vi "User Console View.vi"(8 "error in (no error)":errorcluster, 11 "View Model":T3) -> (0 "error out":errorcluster)   [LabVIEW 2017]
doc: "This console used to select transactions and interact with the ATM controller.\n[Covers: UI2]"
uses:
  View Model/Controls/View Model.ctl
  Error Handler/Controls/Error Model.ctl
  Error Handler/Controls/Error Data.ctl
  Error Handler/Controls/Error Type.ctl
  View Model/Controls/Shared Model.ctl
  Configuration/Controls/Config Model.ctl
  Configuration/Controls/Config CMD.ctl
  Configuration/Controls/Config Data.ctl
  ATM Controller/Controls/Controller Model.ctl
  ATM Controller/Controls/Controller Overhead.ctl
  ATM Controller/Controls/Controller States.ctl
  ATM Controller/Controls/Controller Message Data.ctl
  ATM Controller/Controls/Controller Message Name.ctl
  Controls/User Console - Keypad.ctl
  Controls/User Console - Transactions.ctl
  ATM Controller/Controls/Controller CMD.ctl
panel:
  in  "Card Reader":bool
  in  "Transactions":T1
  in  "Keypad":T2
  # "[Covers: UI2B]"
  # "[Covers: UI2C]"
  # "[Covers: UI2A]"
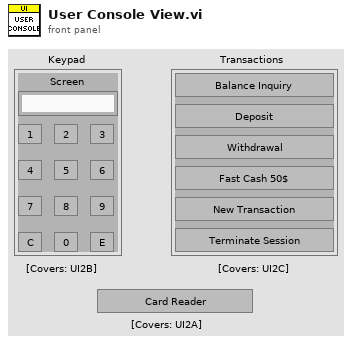
[diagram p1: front panel]
types:
  T1 = typedef "User Console - Transactions.ctl" = cluster{"Balance Inquiry":bool, "Deposit":bool, "Withdrawal":bool, "Fast Cash":bool, "New Transaction":bool, "Terminate":bool}
  T2 = typedef "User Console - Keypad.ctl" = cluster{"Screen":string, "1":bool, "2":bool, "3":bool, "4":bool, "5":bool, "6":bool, "7":bool, "8":bool, "9":bool, "C":bool, "0":bool, "E":bool}
  T3 = typedef "View Model.ctl" = cluster{"Error Model":T4, "Shared Model":T5, "Config Model":T6, "Controller Model":T7}
  T4 = typedef "Error Model.ctl" = cluster{"Error Event":refnum<user-event>}
  T5 = typedef "Shared Model.ctl" = cluster{"Stop Event":refnum<user-event>, "Stop DVR":refnum<data-value>}
  T6 = typedef "Config Model.ctl" = cluster{"Config CMD":refnum<user-event>, "Config Data DVR":refnum<data-value>}
  T7 = typedef "Controller Model.ctl" = cluster{"Controller Overhead DVR":refnum<data-value>, "Deposit Received Change":refnum<user-event>, "Fund Transaction Change":refnum<user-event>, "Card Read Change":refnum<user-event>, "Keypad Change":refnum<user-event>, "Transaction Change":refnum<user-event>, "Controller CMD Change":refnum<user-event>, "Message Change":refnum<user-event>}
  T8 = enum8{"Enabled", "Disabled", "Disabled and Grayed Out"}
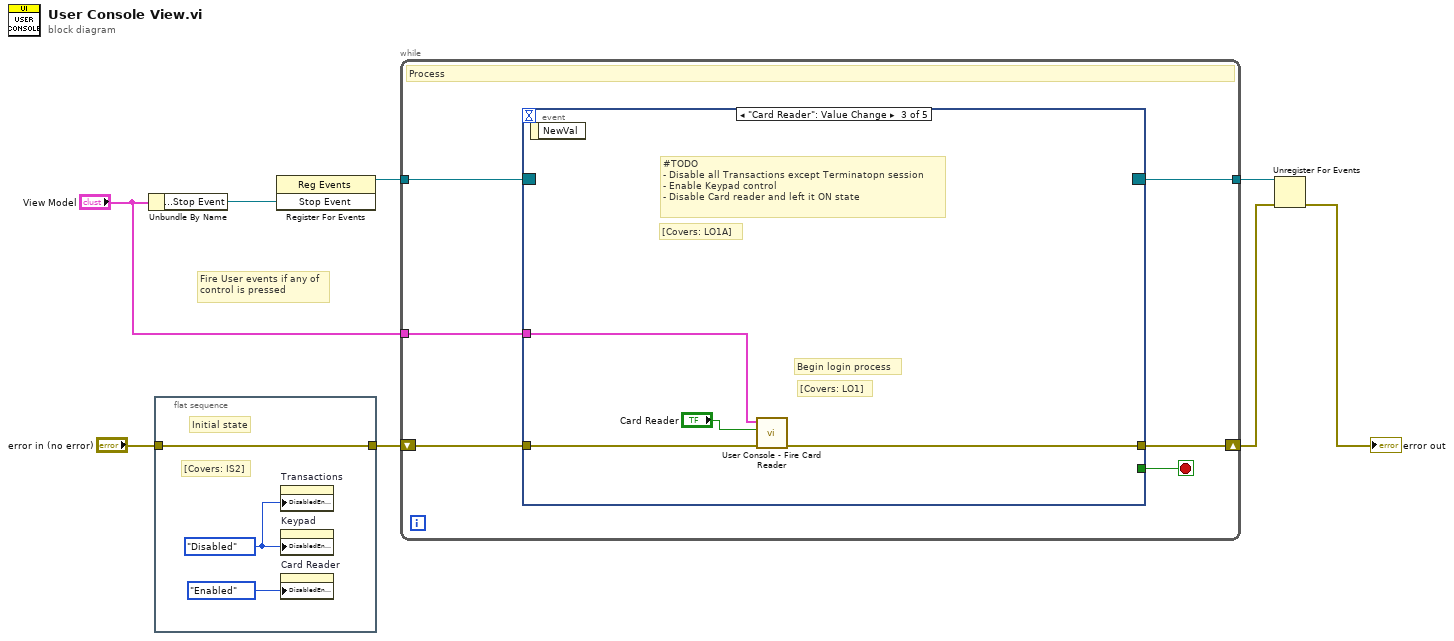
[diagram p0: block diagram]
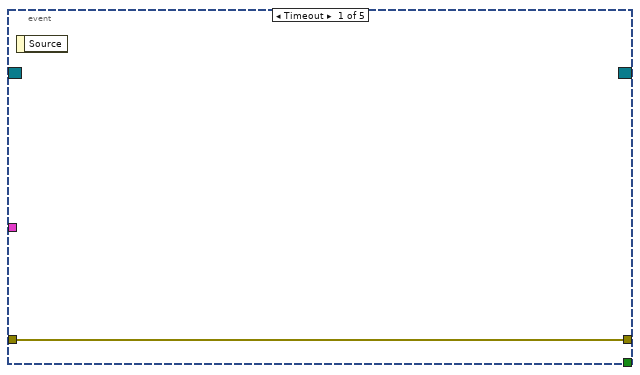
[diagram p2: hidden frame]
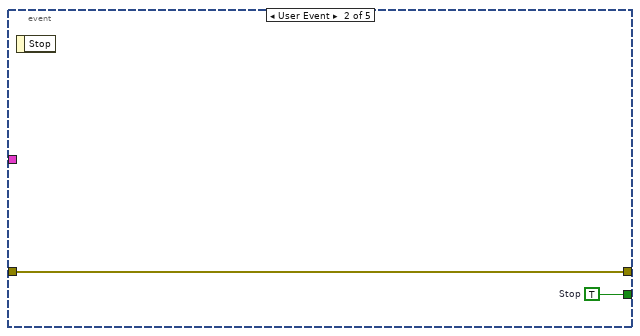
[diagram p3: hidden frame]
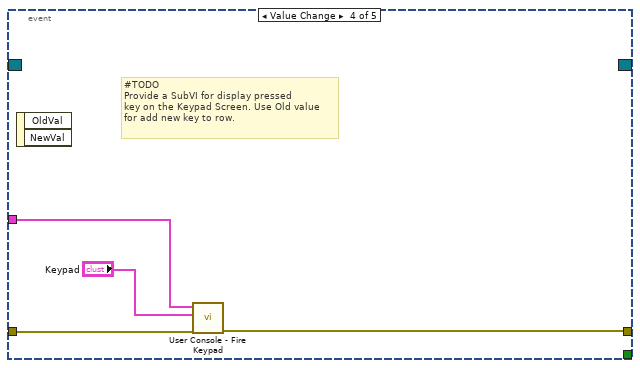
[diagram p4: hidden frame]
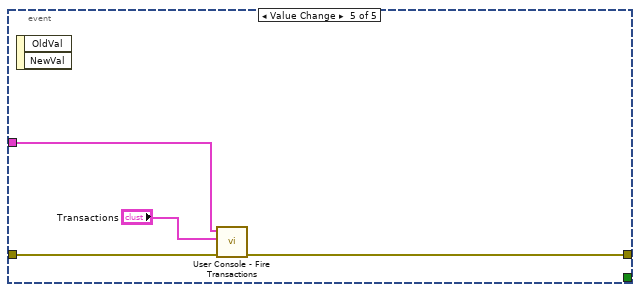
[diagram p5: hidden frame]
diagram:
  # "Fire User events if any of\ncontrol is pressed"
  n1 = Unbundle By Name("View Model") -> ("Shared Model.Stop Event"=w8:refnum<user-event>)
  n2 = flat-sequence {
    tunnel: "error in (no error)" -> [w11]
    tunnel: [w11] -> w1
    frame #0 {
      w9 = T8."Disabled" ("Disabled")
      # "[Covers: IS2]"
      # "Initial state"
      n3 = property on="Transactions" class="Clust"("DisabledEnum"=w9) -> ()  [unwired: 2 in, 2 out]
      n4 = property on="Keypad" class="Clust"("DisabledEnum"=w9) -> ()  [unwired: 2 in, 2 out]
      n5 = property on="Card Reader" class="Bool (strict)"("DisabledEnum"=T8."Enabled" ("Disabled")) -> ()  [unwired: 2 in, 2 out]
    }
  }
  n6 = register-events(w8) -> (reference out=w7:refnum<event-registration>)  [unwired: 2 in, 1 out]
  n7 = while {
    tunnel: w7 -> [w17]
    shift-right: [w14] -> w5
    shift-left: w1 -> [w15]
    tunnel: [w13] -> w6
    tunnel: "View Model" -> [w12]
    stop <- w16 stop-if-true
    # "Process"
    n8 = event shown="[2] \"Card Reader\": Value Change" {
      selector: w17 -> [_ _ _ _ _]
      dyn-events: [_ _ _ _ _] -> w13
      timeout: _ -> [_ _ _ _ _]
      tunnel: [_ w20 _ _ _] -> w16
      tunnel: w15 -> [w18 w19 w24 w28 w32]
      tunnel: [w18 w19 w21 w25 w29] -> w14
      tunnel: w12 -> [_ _ w23 w27 w31]
      event Timeout {
        n9 = event-data() -> ()  [unwired: 1 in, 1 out]
      }
      event User Event {
        w20 = TRUE  # Stop
        n10 = event-data() -> ()  [unwired: 1 in, 1 out]
      }
      event "Card Reader": Value Change {
        # "[Covers: LO1]"
        # "Begin login process"
        # "[Covers: LO1A]"
        # "#TODO\n- Disable all Transactions except Terminatopn session\n- Enable Keypad control\n- Disable Card reader and left it ON state"
        n11 = event-data() -> ()  [unwired: 1 in, 1 out]
        n12 = call "User Console - Fire Card Reader.vi"("error in (no error)"=w24, "Card Reader"="Card Reader", "View Model"=w23) -> ("error out"=w21:errorcluster)  [unwired: 7 in, 1 out]
      }
      event Value Change {
        # "#TODO\nProvide a SubVI for display pressed\nkey on the Keypad Screen. Use Old value\nfor add new key to row."
        n13 = event-data() -> ()  [unwired: 1 in, 2 out]
        n14 = call "User Console - Fire Keypad.vi"("error in (no error)"=w28, "Keypad"="Keypad", "View Model"=w27) -> ("error out"=w25:errorcluster)  [unwired: 7 in, 1 out]
      }
      event Value Change {
        n15 = event-data() -> ()  [unwired: 1 in, 2 out]
        n16 = call "User Console - Fire Transactions.vi"("error in (no error)"=w32, "Transactions"="Transactions", "View Model"=w31) -> ("error out"=w29:errorcluster)  [unwired: 7 in, 1 out]
      }
    }
  }
  n17 = Unregister For Events(event registration refnum=w6, error in=w5) -> (error out=→"error out":errorcluster)
